vi "GetLVDTParameters.vi"(8 "error in (no error)":errorcluster, 11 "Asylum_Driver in":refnum<class "Asylum_Driver.lvclass">) -> (0 "error out":errorcluster, 2 "LVDT Parameters":T1, 3 "Asylum_Driver out":refnum<class "Asylum_Driver.lvclass">)   [LabVIEW 2019, in "Asylum_Driver.lvclass"]
uses:
  Asylum_Driver.lvclass
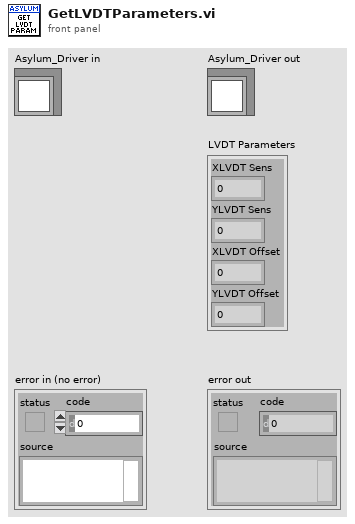
[diagram p1: front panel]
types:
  T1 = cluster{"XLVDT Sens":dbl, "YLVDT Sens":dbl, "XLVDT Offset":dbl, "YLVDT Offset":dbl}
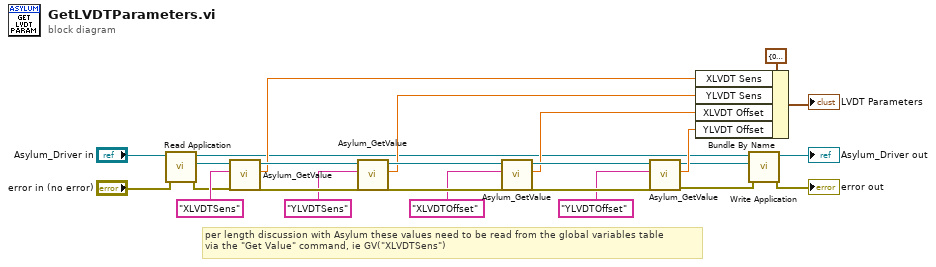
[diagram p0: block diagram]
diagram:
  # "per length discussion with Asylum these values need to be read from the global variables table\nvia the \"Get Value\" command, ie GV(\"XLVDTSens\")"
  n1 = call-dynamic "Read Application.vi"("error in (no error)"="error in (no error)", "Asylum_Driver in"="Asylum_Driver in") -> ("error out"=w4:errorcluster, "Application"=w8:refnum<k7>, "Asylum_Driver out"=w10:refnum<class "Asylum_Driver.lvclass">)  [unwired: 7 in]
  n2 = call <userlib>:"Asylum_GetValue.vi"("error in (no error)"=w4, "Value"="XLVDTSens", "Application"=w8) -> ("error out"=w23:errorcluster, "Value"=w15:dbl, "Application"=w24:refnum<k7>)  [unwired: 6 in]
  n3 = call <userlib>:"Asylum_GetValue.vi"("error in (no error)"=w23, "Value"="YLVDTSens", "Application"=w24) -> ("error out"=w21:errorcluster, "Value"=w16:dbl, "Application"=w22:refnum<k7>)  [unwired: 6 in]
  n4 = call <userlib>:"Asylum_GetValue.vi"("error in (no error)"=w21, "Value"="XLVDTOffset", "Application"=w22) -> ("error out"=w19:errorcluster, "Value"=w17:dbl, "Application"=w20:refnum<k7>)  [unwired: 6 in]
  n5 = call <userlib>:"Asylum_GetValue.vi"("error in (no error)"=w19, "Value"="YLVDTOffset", "Application"=w20) -> ("error out"=w7:errorcluster, "Value"=w18:dbl, "Application"=w9:refnum<k7>)  [unwired: 6 in]
  n6 = Bundle By Name(cluster=T1 {"XLVDT Sens"=0.0, "YLVDT Sens"=0.0, "XLVDT Offset"=0.0, "YLVDT Offset"=0.0} ("LVDT Parameters"), "XLVDT Sens"=w15, "YLVDT Sens"=w16, "XLVDT Offset"=w17, "YLVDT Offset"=w18) -> (→"LVDT Parameters":T1)
  n7 = call-dynamic "Write Application.vi"("error in (no error)"=w7, "Application"=w9, "Asylum_Driver in"=w10) -> ("error out"=→"error out":errorcluster, "Asylum_Driver out"=→"Asylum_Driver out":refnum<class "Asylum_Driver.lvclass">)  [unwired: 7 in]
